vi "get tone info.vi"(8 "error in (no error)":errorcluster, 10 "Expected Frequency":dbl, 11 "time signal in":waveform(dbl)) -> (0 "error out":errorcluster, 2 "Amplitude":dbl, 3 "Dominant Frequency":dbl)   [LabVIEW 2011]
uses:
  <vilib>/measure/matone.llb/Extract Single Tone Information 1 Chan.vi
  <vilib>/measure/NI_MAPro.lvlib
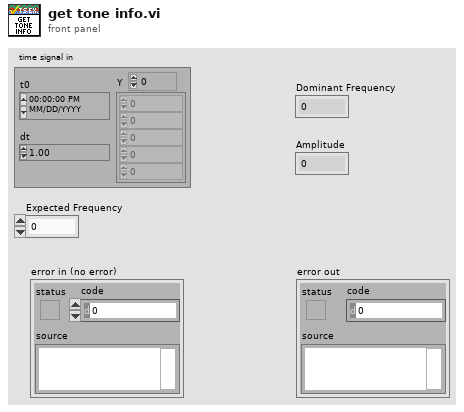
[diagram p1: front panel]
types:
  T1 = cluster{"Expected Frequency":dbl, "search (+/- % of Fsampl.)":dbl}
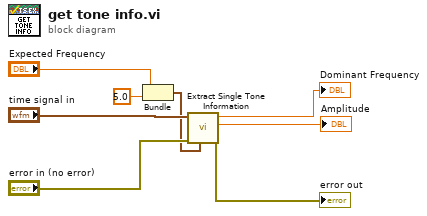
[diagram p0: block diagram]
diagram:
  n1 = Bundle("Expected Frequency"="Expected Frequency", "search (+/- % of Fsampl.)"=5.0) -> (w1:T1)  [unwired: 1 in]
  n2 = call-poly <vilib>:"Extract Single Tone Information.vi"("advanced search"=w1, "error in (no error)"="error in (no error)", "time signal in"="time signal in") -> ("error out"=→"error out":errorcluster, "detected amplitude"=→"Amplitude":dbl, "detected frequency"=→"Dominant Frequency":dbl)  [unwired: 3 in, 3 out]
